vi "Convert dBFS to V.vi"(1 "Amplitude (dBFS)":dbl) -> (0 "Amplitude (V)":dbl)   [LabVIEW 2021, in "IMD_Audio ADC.lvlib"]
uses:
  IMD_Audio ADC.lvlib
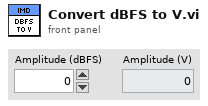
[diagram p1: front panel]
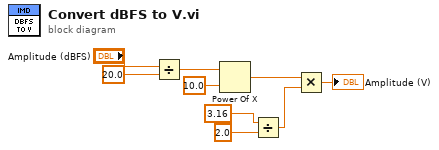
[diagram p0: block diagram]
diagram:
  n1 = Divide(x="Amplitude (dBFS)", y=20.0) -> (x/y=w9:dbl)
  n2 = Power Of X(1:10.0 ("x"), 2:w9) -> (0:w5:dbl)
  n3 = Divide(x=3.16, y=2.0) -> (x/y=w4:dbl)
  n4 = Multiply(x=w5, y=w4) -> (x*y=→"Amplitude (V)":dbl)
